vi "Main.vi"() -> ()   [LabVIEW 2017]
uses:
  <vilib>/NI/PowerElectronicsControl/ScaleAndLimit/Interface/ScaleAndLimitInterface.lvlib
  <vilib>/NI/PowerElectronicsControl/ScaleAndLimit/Interface/Configuration.ctl
  <vilib>/rvi/interface/nirviReadWriteControl/nirviReadWriteControl.xnode
  <vilib>/rvi/interface/nirviCloseFPGA/nirviCloseFPGA.xnode
  <instrlib>/_niInstr/FIFO Register Bus/v1/Host/niInstr FIFO Register Bus v1 Host.lvclass
  <instrlib>/_niInstr/Instruction Framework/v1/Host/Subsystem Map/niInstr Subsystem Map v1 Host.lvclass
  <vilib>/rvi/interface/nirviOpenFPGA/nirviOpenFPGA.xnode
  <vilib>/NI/PowerElectronicsControl/WaveformAcq/RT/WaveformTask.lvclass
  <vilib>/NI/PowerElectronicsControl/BufferLogging/BufferLogging.lvlib
  <vilib>/NI/PowerElectronicsControl/BufferLogging/BufferConfig.ctl
  <vilib>/rvi/interface/nirviMethod/nirviMethod.xnode
  <vilib>/rvi/interface/nirviMethod/StockFPGA_InlinedMethodWaitForSingleIRQ.vi
  <vilib>/FPGAPlugInAG/Dynamic/niLvFpga_WaitOnIrq_Dynamic.vi
  NiFpgaLv.dll
  <vilib>/Utility/error.llb/Error Cluster From Error Code.vi
  <vilib>/rvi/interface/Simulation/niFpgaSimulationCallBeginRW.vi
  <vilib>/rvi/errors/niLvFpgaAdjustHostInterfaceError.vi
  <vilib>/FPGAPlugInAG/Dynamic/niLvFpga_AcknowledgeIrq_Dynamic.vi
  <vilib>/FPGAPlugInAG/Dynamic/niLvFpga_Close_Dynamic.vi
  <vilib>/NI/PowerElectronicsControl/WaveformAcq/RT/ReadInterleaved.vi
  C:/Program Files (x86)/National Instruments/LabVIEW 2017/instr.lib/_niInstr/Instruction Framework/v1/Host/Instruction Target/niInstr Instruction Target v1 Host.lvclass
  FPGA Bitfiles/DevelopmentTempl_FPGATarget_Firmware_p1stBaQsGw8.lvbitx
  FPGA/Firmware.vi
  <vilib>/FPGAPlugInAG/sbRIO-9607/niLvFpga_Open_sbRIO-9607.vi
  <vilib>/rvi/interface/common/dynamic/niFpgaDynamicAddResources.vi
panel:
  out "snapshot":waveform(sgl)[](graph)
  in  "Update Time (s)":dbl=5.0 caption="Time Target (s)" min=1.0
  in  "ManualTrigger":bool
  out "Limits":string
  out "SimultaneousAILoopRate":u32
  out "SimultaneousAI":sgl[](array[numeric])
  in  "clearLimits":bool
  in  "stop":bool
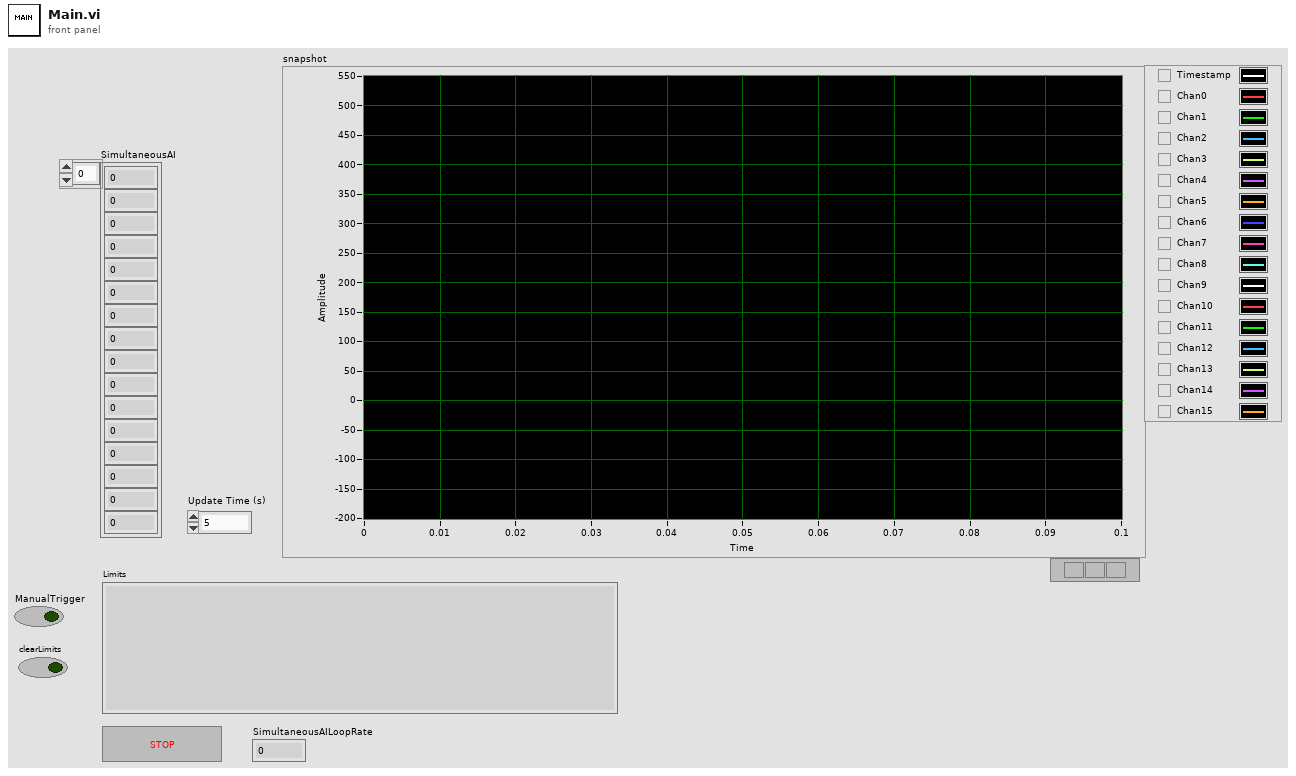
[diagram p1: front panel]
types:
  T1 = typedef "BufferLogging.lvlib/BufferConfig.ctl" = cluster{"Channels":string[], "pretriggerTime_sec":dbl, "posttriggerTime_sec":dbl, "BlockSizePerChannel":i32, "SampleRate_Hz":dbl, "decimation factor":i32, "logDirectory":string, "logPrefix":string, "max files":i32}
  T2 = typedef "ScaleAndLimitInterface.lvlib/Configuration.ctl" = cluster{"Name":string, "M":dbl, "B":i16, "HighLimit":dbl, "LowLimit":dbl, "LimitsEnabled":bool}
  T3 = typedef "BufferLogging.lvlib/Buffers.ctl" = cluster{"Channels":string[], "PosttriggerBuffer":refnum<queue>, "PretriggerBuffer":refnum<queue>, "BlockSizePerChannel":i32, " logging semaphore":T4, "Log refnum":refnum<k34>, "snapshotBuffer":refnum<data-value>, "logDirectory":path, "logPrefix":string, "decimation factor":i32, "max files":i32, "SampleRate":dbl}
  T4 = typedef "Semaphore RefNum" = refnum<k1>
  T5 = typedef "ScaleAndLimitInterface.lvlib/Interface.ctl" = cluster{"instruction target":refnum<class "niInstr Instruction Target v1 Host.lvclass">, "ScalingAndLimitsContext":refnum<class "niInstr Instruction Framework Context v1 Host.lvclass">, "Configuration":T2[]}
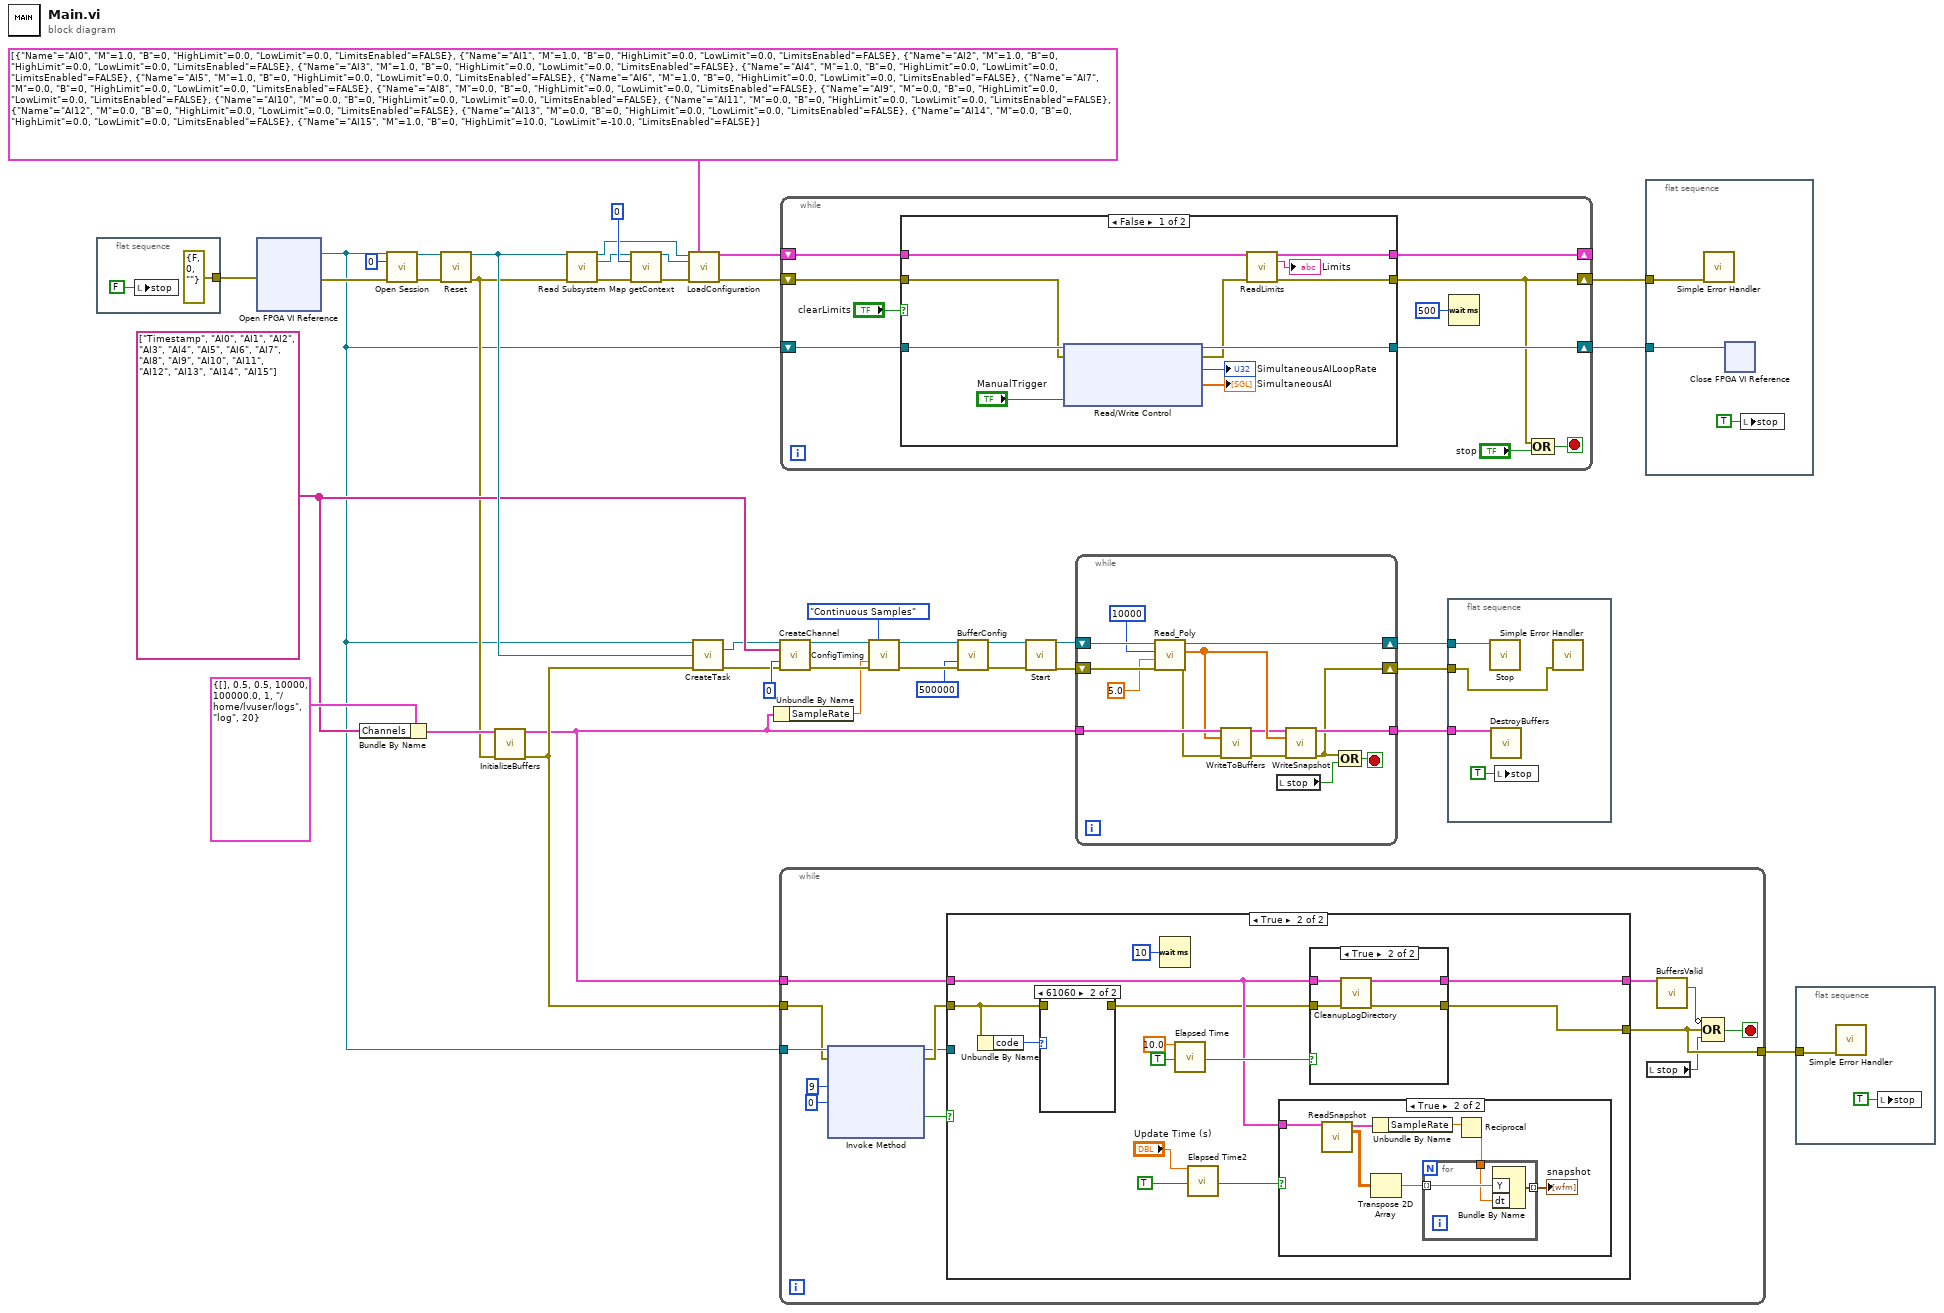
[diagram p0: block diagram]
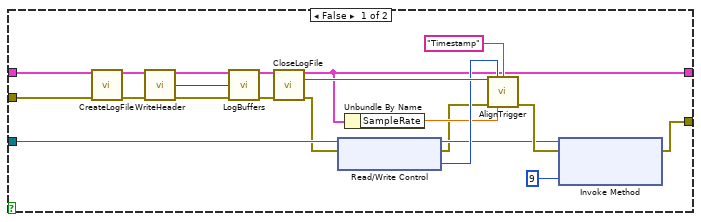
[diagram p2: hidden frame]
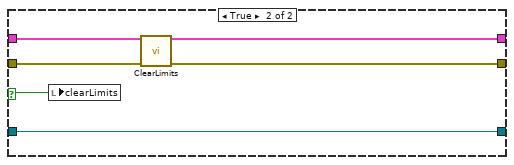
[diagram p6: hidden frame]
diagram:
  w29 = string[] ["Timestamp", "AI0", "AI1", "AI2", "AI3", "AI4", "AI5", "AI6", "AI7", "AI8", "AI9", "AI10", "AI11", "AI12", "AI13", "AI14", "AI15"] ("Chan Name Array")
  n1 = flat-sequence {
    tunnel: [errorcluster {"status"=FALSE, "code"=0, "source"=""} ("error in")] -> w26
    frame #0 {
      n2 = local write "stop"(FALSE ("stop")) -> ()
    }
  }
  n3 = xnode "Open FPGA VI Reference"("error in"=w26) -> ("FPGA VI Reference Out"=w24:refnum<k20>, "error out"=w32:errorcluster)  [unwired: 1 in]
  n4 = Bundle By Name(cluster=T1 {"Channels"=[], "pretriggerTime_sec"=0.5, "posttriggerTime_sec"=0.5, "BlockSizePerChannel"=10000, "SampleRate_Hz"=100000.0, "decimation factor"=1, "logDirectory"="/home/lvuser/logs", "logPrefix"="log", "max files"=20} ("BufferConfig"), "Channels"=w29) -> (w28:T1)
  n5 = call <instrlib>:"Open Session.vi"("fpga ref"=w24, "bus instance"=u32 0, "error in"=w32) -> ("session out"=w35:refnum<class "niInstr FIFO Register Bus v1 Host.lvclass">, "error out"=w36:errorcluster)  [unwired: 11 in]
  n6 = call-dynamic "Reset.vi"("session in"=w35, "error in"=w36) -> ("session out"=w31:refnum<class "niInstr FIFO Register Bus v1 Host.lvclass">, "error out"=w27:errorcluster)  [unwired: 12 in]
  n7 = call <vilib>:"InitializeBuffers.vi"("BufferConfig"=w28, "error in (no error)"=w27) -> ("Buffers"=w22:T3, "error out"=w23:errorcluster)  [unwired: 12 in]
  n8 = call <instrlib>:"Read Subsystem Map.vi"("instruction target in"=w31, "error in"=w27) -> ("instruction target out"=w2:refnum<class "niInstr FIFO Register Bus v1 Host.lvclass">, "subsystem map"=w1:refnum<class "niInstr Subsystem Map v1 Host.lvclass">, "error out"=w34:errorcluster)  [unwired: 11 in]
  n9 = call <vilib>:"getContext.vi"("subsystemMap"=w1, "instance"=u8 0, "error in"=w34) -> ("ScalingAndLimitsContext"=w3:refnum<class "niInstr Instruction Framework Context v1 Host.lvclass">, "error out"=w42:errorcluster)  [unwired: 11 in]
  n10 = call <vilib>:"LoadConfiguration.vi"("instruction target in"=w2, "Configuration"=T2[] [{"Name"="AI0", "M"=1.0, "B"=0, "HighLimit"=0.0, "LowLimit"=0.0, "LimitsEnabled"=FALSE}, {"Name"="AI1", "M"=1.0, "B"=0, "HighLimit"=0.0, "LowLimit"=0.0, "LimitsEnabled"=FALSE}, {"Name"="AI2", "M"=1.0, "B"=0, "HighLimit"=0.0, "LowLimit"=0.0, "LimitsEnabled"=FALSE}, {"Name"="AI3", "M"=1.0, "B"=0, "HighLimit"=0.0, "LowLimit"=0.0, "LimitsEnabled"=FALSE}, {"Name"="AI4", "M"=1.0, "B"=0, "HighLimit"=0.0, "LowLimit"=0.0, "LimitsEnabled"=FALSE}, {"Name"="AI5", "M"=1.0, "B"=0, "HighLimit"=0.0, "LowLimit"=0.0, "LimitsEnabled"=FALSE}, {"Name"="AI6", "M"=1.0, "B"=0, "HighLimit"=0.0, "LowLimit"=0.0, "LimitsEnabled"=FALSE}, {"Name"="AI7", "M"=0.0, "B"=0, "HighLimit"=0.0, "LowLimit"=0.0, "LimitsEnabled"=FALSE}, {"Name"="AI8", "M"=0.0, "B"=0, "HighLimit"=0.0, "LowLimit"=0.0, "LimitsEnabled"=FALSE}, {"Name"="AI9", "M"=0.0, "B"=0, "HighLimit"=0.0, "LowLimit"=0.0, "LimitsEnabled"=FALSE}, {"Name"="AI10", "M"=0.0, "B"=0, "HighLimit"=0.0, "LowLimit"=0.0, "LimitsEnabled"=FALSE}, {"Name"="AI11", "M"=0.0, "B"=0, "HighLimit"=0.0, "LowLimit"=0.0, "LimitsEnabled"=FALSE}, {"Name"="AI12", "M"=0.0, "B"=0, "HighLimit"=0.0, "LowLimit"=0.0, "LimitsEnabled"=FALSE}, {"Name"="AI13", "M"=0.0, "B"=0, "HighLimit"=0.0, "LowLimit"=0.0, "LimitsEnabled"=FALSE}, {"Name"="AI14", "M"=0.0, "B"=0, "HighLimit"=0.0, "LowLimit"=0.0, "LimitsEnabled"=FALSE}, {"Name"="AI15", "M"=1.0, "B"=0, "HighLimit"=10.0, "LowLimit"=-10.0, "LimitsEnabled"=FALSE}], "ScalingAndLimitsContext"=w3, "error in (no error)"=w42) -> ("Interface"=w39:T5, "error out"=w38:errorcluster)  [unwired: 10 in]
  n11 = call <vilib>:"CreateTask.vi"("FPGA Ref in"=w24, "session in"=w31, "error in"=w23) -> ("Task out"=w9:refnum<class "WaveformTask.lvclass">, "error out"=w8:errorcluster)  [unwired: 9 in, 2 out]
  n12 = Unbundle By Name(w22) -> ("SampleRate"=w5:dbl)
  n13 = call <vilib>:"CreateChannel.vi"("task in"=w9, "Chan Name Array"=w29, "instance"=u8 0, "error in"=w8) -> ("Task out"=w10:refnum<class "WaveformTask.lvclass">, "error out"=w19:errorcluster)  [unwired: 10 in]
  n14 = while {
    tunnel: w23 -> [w49]
    tunnel: w22 -> [w57]
    tunnel: w24 -> [w53]
    tunnel: [w46] -> w21
    stop <- w55 stop-if-true
    n15 = xnode "Invoke Method"("FPGA VI Reference In"=w53, "error in"=w49, "IRQ Number(s)"=9, "Timeout (ms)"=0) -> ("FPGA VI Reference Out"=w47:refnum<k20>, "error out"=w48:errorcluster, "Timed Out"=w50:bool)  [unwired: 1 out]
    n16 = case shown="True" w50 {
      tunnel: w48 -> [w78 w81]
      tunnel: w57 -> [w77 w82]
      tunnel: [w62 w86] -> w56
      tunnel: [w68 w87] -> w46
      tunnel: w47 -> [w64 _]
      frame False {
        n17 = call <vilib>:"CreateLogFile.vi"("Buffers in"=w77, "error in (no error)"=w78) -> ("Buffers out"=w76:T3, "error out"=w75:errorcluster)  [unwired: 12 in]
        n18 = call <vilib>:"WriteHeader.vi"("Buffers in"=w76, "error in (no error)"=w75) -> ("Buffers out"=w74:T3, "numOfChannels"=w72:i32, "error out"=w73:errorcluster)  [unwired: 11 in]
        n19 = call <vilib>:"LogBuffers.vi"("Buffers in"=w74, "numOfChannels"=w72, "error in (no error)"=w73) -> ("Buffers out"=w71:T3, "error out"=w70:errorcluster)  [unwired: 11 in]
        n20 = call <vilib>:"CloseLogFile.vi"("Buffers in"=w71, "error in (no error)"=w70) -> ("Buffers out"=w62:T3, "log path out"=w67:path, "error out"=w60:errorcluster)  [unwired: 11 in]
        n21 = xnode "Read/Write Control"("FPGA VI Reference In"=w64, "error in"=w60) -> ("FPGA VI Reference Out"=w59:refnum<k20>, "error out"=w58:errorcluster, "TriggerTimestamp"=w63:i32)
        n22 = Unbundle By Name(w62) -> ("SampleRate"=w61:dbl)
        n23 = call <vilib>:"AlignTrigger.vi"("log path in"=w67, "triggerTimestamp"=w63, "alignmentChannel"="Timestamp", "error in (no error)"=w58, "AcqRate"=w61) -> ("error out"=w65:errorcluster)  [unwired: 9 in, 1 out]
        n24 = xnode "Invoke Method"("FPGA VI Reference In"=w59, "error in"=w65, "IRQ Number(s)"=9) -> ("error out"=w68:errorcluster)  [unwired: 1 out]
      }
      frame True {
        n25 = Unbundle By Name(w81) -> ("code"=w80:i32)
        n26 = case shown="61060" w80 {
          tunnel: w81 -> [w92 _]
          tunnel: [w92 _] -> w79
          frame 0, Default {
          }
          frame 61060 {
          }
        }
        n27 = Wait (ms)(milliseconds to wait=u32 10) -> ()  [unwired: 1 out]
        n28 = call "Elapsed Time"("Time Target (s)"=10.0, "Auto Reset"=TRUE) -> ("Time has Elapsed"=w88:bool)  [unwired: 10 in, 7 out]
        n29 = call "Elapsed Time2"("Time Target (s)"="Update Time (s)", "Auto Reset"=TRUE) -> ("Time has Elapsed"=w83:bool)  [unwired: 10 in, 7 out]
        n30 = case shown="True" w83 {
          tunnel: w82 -> [_ w93]
          frame False {
          }
          frame True {
            n31 = call <vilib>:"ReadSnapshot.vi"("Buffers in"=w93) -> ("Buffers out"=w96:T3, "snapshot"=w99:sgl[][])  [unwired: 12 in, 1 out]
            n32 = Transpose 2D Array(2D array=w99) -> (transposed array=w98:sgl[][])
            n33 = Unbundle By Name(w96) -> ("SampleRate"=w95:dbl)
            n34 = Reciprocal(x=w95) -> (1/x=w94:dbl)
            n35 = for {
              tunnel: w98 -> [w102] mode=indexing
              tunnel: [w101] -> w97 mode=indexing
              tunnel: w94 -> [w100]
              n36 = Bundle By Name("Y"=w102, "dt"=w100) -> (w101:waveform(sgl))  [unwired: 1 in]
            }
            "snapshot" <- w97
          }
        }
        n37 = case shown="True" w88 {
          tunnel: w79 -> [w104 w108]
          tunnel: [w104 w107] -> w87
          tunnel: w82 -> [w103 w106]
          tunnel: [w103 w105] -> w86
          frame False {
          }
          frame True {
            n38 = call <vilib>:"CleanupLogDirectory.vi"("BuffersIn"=w106, "error in"=w108) -> ("BuffersOut"=w105:T3, "error out"=w107:errorcluster)  [unwired: 12 in]
          }
        }
      }
    }
    n39 = local read "stop"() -> (w45:bool)
    n40 = call <vilib>:"BuffersValid.vi"("Buffers in"=w56) -> ("valid"=w54:bool)  [unwired: 13 in, 1 out]
    n41 = Compound Arithmetic op=OR(invert w54, w46, w45) -> (w55:bool)
  }
  n42 = while {
    shift-right: [w112] -> _
    shift-left: w39 -> [w118]
    shift-right: [w110] -> w25
    shift-left: w38 -> [w117]
    shift-right: [w113] -> w37
    shift-left: w24 -> [w114]
    stop <- w111 stop-if-true
    n43 = case shown="False" "clearLimits" {
      selector: "clearLimits" -> [_ w130]
      tunnel: w118 -> [w126 w135]
      tunnel: w117 -> [w128 w134]
      tunnel: [w125 w133] -> w112
      tunnel: [w124 w132] -> w110
      tunnel: w114 -> [w129 w131]
      tunnel: [w127 w131] -> w113
      frame False {
        n44 = xnode "Read/Write Control"("FPGA VI Reference In"=w129, "error in"=w128, "ManualTrigger"="ManualTrigger") -> ("FPGA VI Reference Out"=w127:refnum<k20>, "error out"=w122:errorcluster, "SimultaneousAILoopRate"=→"SimultaneousAILoopRate":u32, "Simultaneous_AI"=→"SimultaneousAI":sgl[])
        n45 = call <vilib>:"ReadLimits.vi"("Interface in"=w126, "error in (no error)"=w122) -> ("Interface out"=w125:T5, "Limits"=→"Limits":string, "error out"=w124:errorcluster)  [unwired: 11 in]
      }
      frame True {
        n46 = local write "clearLimits"(w130) -> ()
        n47 = call <vilib>:"ClearLimits.vi"("Interface in"=w135, "error in (no error)"=w134) -> ("Interface out"=w133:T5, "error out"=w132:errorcluster)  [unwired: 12 in]
      }
    }
    n48 = Wait (ms)(milliseconds to wait=u32 500) -> ()  [unwired: 1 out]
    n49 = Compound Arithmetic op=OR(w110, "stop") -> (w111:bool)
  }
  n50 = call <vilib>:"ConfigTiming.vi"("Task in"=w10, "Sample Mode"=enum16{"Finite Samples", "Continuous Samples"}."Continuous Samples", "Sample Rate"=w5, "error in (no error)"=w19) -> ("Task out"=w17:refnum<class "WaveformTask.lvclass">, "error out"=w16:errorcluster)  [unwired: 9 in, 1 out]
  n51 = call <vilib>:"BufferConfig.vi"("WaveformTask in"=w17, "Buffer Size [Samps per Chan]"=500000, "error in (no error)"=w16) -> ("WaveformTask out"=w14:refnum<class "WaveformTask.lvclass">, "error out"=w13:errorcluster)  [unwired: 10 in, 1 out]
  n52 = call <vilib>:"Start.vi"("WaveformTask in"=w14, "error in (no error)"=w13) -> ("WaveformTask out"=w12:refnum<class "WaveformTask.lvclass">, "error out"=w11:errorcluster)  [unwired: 12 in]
  n53 = while {
    shift-right: [w141] -> w4
    shift-left: w11 -> [w148]
    shift-right: [w147] -> w7
    shift-left: w12 -> [w149]
    tunnel: w22 -> [w146]
    tunnel: [w144] -> w6
    stop <- w140 stop-if-true
    n54 = call-poly <vilib>:"Read_Poly.vi"("error in"=w148, "Timeout (s)"=5.0, "Samps Read per Chan"=10000, "Task in"=w149) -> ("error out"=w136:errorcluster, "Data"=w145:sgl[], "Task out"=w147:refnum<class "WaveformTask.lvclass">)  [unwired: 4 in, 1 out]
    n55 = call <vilib>:"WriteToBuffers.vi"("Buffers in"=w146, "Data"=w145, "error in (no error)"=w136) -> ("Buffers out"=w142:T3, "error out"=w143:errorcluster)  [unwired: 11 in]
    n56 = local read "stop"() -> (w139:bool)
    n57 = call <vilib>:"WriteSnapshot.vi"("Buffers in"=w142, "Snapshot"=w145, "error in (no error)"=w143) -> ("Buffers out"=w144:T3, "error out"=w141:errorcluster)  [unwired: 11 in]
    n58 = Compound Arithmetic op=OR(w141, w139) -> (w140:bool)
  }
  n59 = flat-sequence {
    tunnel: w7 -> [w153]
    tunnel: w6 -> [w152]
    tunnel: w4 -> [w150]
    frame #0 {
      n60 = call <vilib>:"Stop.vi"("WaveformTask in"=w153) -> ()  [unwired: 9 in, 2 out]
      n61 = call <vilib>:"DestroyBuffers.vi"("Buffers"=w152) -> ()  [unwired: 14 in, 1 out]
      n62 = local write "stop"(TRUE ("stop")) -> ()
      n63 = call <vilib>:"Simple Error Handler.vi"("error in (no error)"=w150) -> ()  [unwired: 4 in, 5 out]
    }
  }
  n64 = flat-sequence {
    tunnel: w37 -> [w156]
    tunnel: w25 -> [w154]
    frame #0 {
      n65 = call <vilib>:"Simple Error Handler.vi"("error in (no error)"=w154) -> ()  [unwired: 4 in, 5 out]
      n66 = xnode "Close FPGA VI Reference"("FPGA VI Reference In"=w156) -> ()  [unwired: 1 in, 1 out]
      n67 = local write "stop"(TRUE ("stop")) -> ()
    }
  }
  n68 = flat-sequence {
    tunnel: w21 -> [w157]
    frame #0 {
      n69 = call <vilib>:"Simple Error Handler.vi"("error in (no error)"=w157) -> ()  [unwired: 4 in, 5 out]
      n70 = local write "stop"(TRUE ("stop")) -> ()
    }
  }
